vi "loginProgram.vi"() -> ()   [LabVIEW 2014]
panel:
  in  "退出 2":bool
  in  "登录 2":bool
  in  "密码":string
  in  "用户名":string
  in  "错误输入（无错误）":errorcluster
  out "password":string
  out "username":string
  # "用户登录"
  # "用户名"
  # "密码"
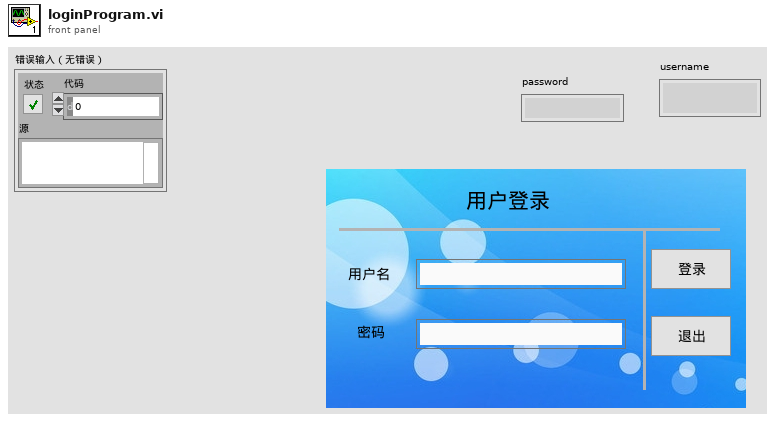
[diagram p1: front panel]
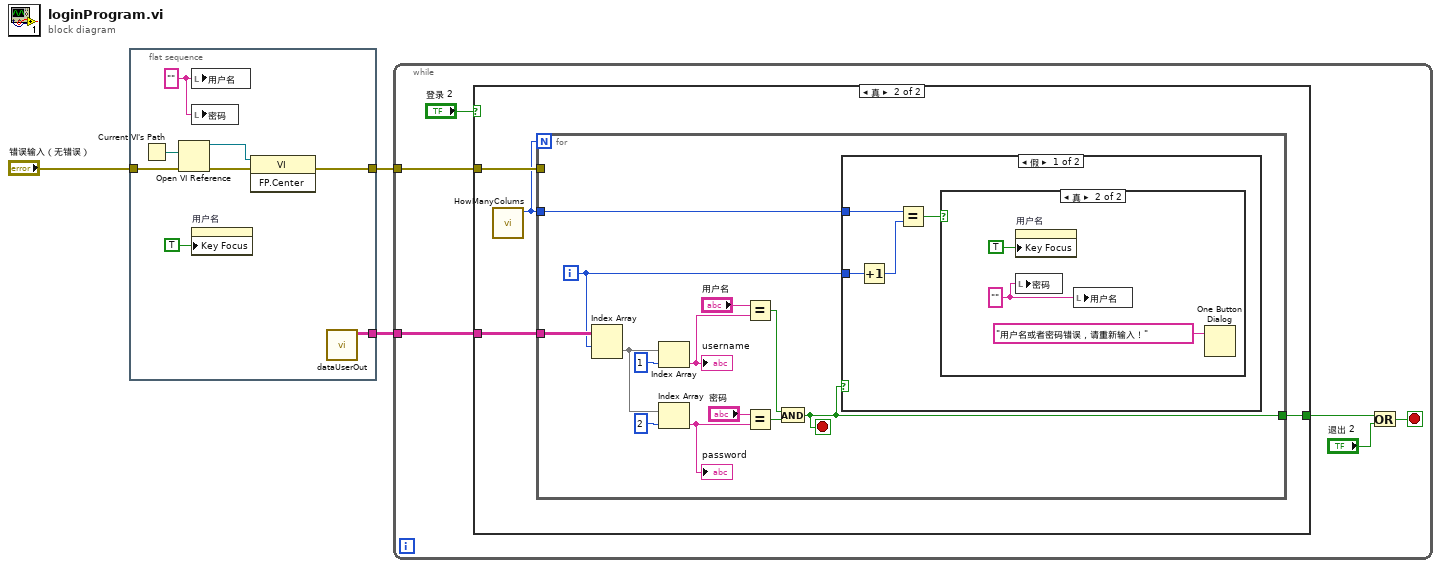
[diagram p0: block diagram]
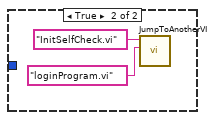
[diagram p4: hidden frame]
diagram:
  n1 = flat-sequence {
    tunnel: [w11] -> w3
    tunnel: "错误输入（无错误）" -> [w7]
    tunnel: [w5] -> w1
    frame #0 {
      w8 = ""
      n2 = Current VI's Path() -> (path=w9:path)
      n3 = Open VI Reference(vi path=w9, error in (no error)=w7) -> (vi reference=w10:refnum<vi>, error out=w6:errorcluster)  [unwired: 4 in]
      n4 = local write "用户名"(w8) -> ()
      n5 = local write "密码"(w8) -> ()
      n6 = property on="用户名" class="Str"("Key Focus"=TRUE ("键选中")) -> ()  [unwired: 2 in, 2 out]
      n7 = invoke class="VI" method="FP.Center"(reference=w10, error in=w6) -> (error out=w5:errorcluster)  [unwired: 1 in, 2 out]
      n8 = call "dataUserOut.vi"() -> ("Data"=w11:string[][])  [unwired: 10 in, 1 out]
    }
  }
  n9 = while {
    tunnel: w3 -> [w17]
    tunnel: w1 -> [w16]
    stop <- w14 stop-if-true
    n10 = case shown="真" "登录 2" {
      tunnel: w17 -> [_ w20]
      tunnel: w16 -> [_ w21]
      tunnel: [_ w19] -> w15
      frame False {
      }
      frame True {
        n11 = call "HowManyColums.vi"() -> ("数目"=w18:i32)  [unwired: 10 in, 1 out]
        n12 = for {
          N: w18 -> [_]
          tunnel: w21 -> [_]
          tunnel: w20 -> [w25]
          tunnel: [w22] -> w19
          tunnel: w18 -> [w23]
          i -> [w24]
          stop <- w22 stop-if-true
          n13 = Index Array(array=w25, index (row)=w24) -> (element=w34:string[])  [unwired: 1 in]
          n14 = Index Array(array=w34, index=1 ("索引 (行)")) -> (element=w31:string)
          "username" <- w31
          n15 = Index Array(array=w34, index=2 ("索引 (行)")) -> (element=w29:string)
          "password" <- w29
          n16 = Equal?(x="用户名", y=w31) -> (x = y?=w30:bool)
          n17 = Equal?(x="密码", y=w29) -> (x = y?=w28:bool)
          n18 = And(x=w30, y=w28) -> (x .and. y?=w22:bool)
          n19 = case shown="假" w22 {
            tunnel: w24 -> [w38 _]
            tunnel: w23 -> [w35 _]
            frame False {
              n20 = Increment(x=w38) -> (x+1=w37:i32)
              n21 = Equal?(x=w35, y=w37) -> (x = y?=w36:bool)
              n22 = case shown="真" w36 {
                frame False {
                }
                frame True {
                  w39 = ""
                  n23 = property on="用户名" class="Str"("Key Focus"=TRUE ("键选中")) -> ()  [unwired: 2 in, 2 out]
                  n24 = local write "密码"(w39) -> ()
                  n25 = local write "用户名"(w39) -> ()
                  n26 = One Button Dialog(message="用户名或者密码错误，请重新输入！" ("消息")) -> ()  [unwired: 1 in, 1 out]
                }
              }
            }
            frame True {
              n27 = call "JumpToAnotherVI.vi"("要关闭的VI"="loginProgram.vi", "要打开的VI"="InitSelfCheck.vi") -> ()  [unwired: 9 in, 1 out]
            }
          }
        }
      }
    }
    n28 = Or(x=w15, y="退出 2") -> (x .or. y?=w14:bool)
  }
